vi "Process Standard Output.vi"(8 "error in (no error)":errorcluster, 11 "InsightCM Console Wrapper in":refnum<class "InsightCM Console Wrapper.lvclass">) -> (0 "error out":errorcluster, 2 "Command Output":string, 3 "InsightCM Console Wrapper out":refnum<class "InsightCM Console Wrapper.lvclass">)   [LabVIEW 2020, in "InsightCM Console Wrapper.lvclass"]
uses:
  InsightCM Console Wrapper.lvclass
  C:/Users/fflores/Documents/GitHub Projects/LabVIEW-CLI-Wrapper/Console Wrapper/Console Wrapper.lvclass
  Console Wrapper/Read Standard Output.vi
  <vilib>/Utility/error.llb/Error Cluster From Error Code.vi
  <vilib>/ErrorRing/Error Ring.xnode
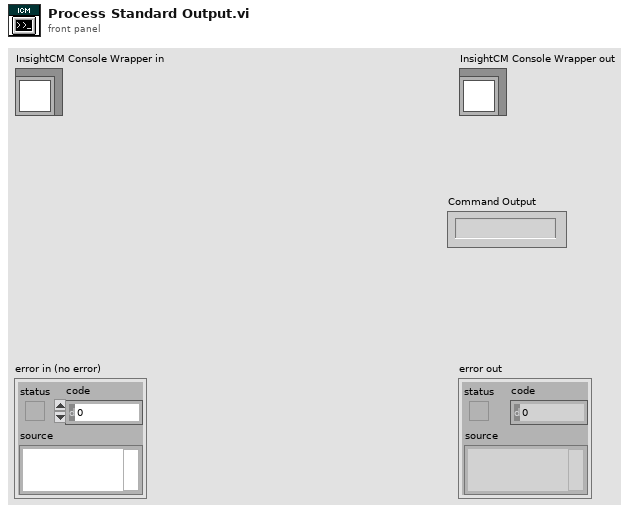
[diagram p1: front panel]
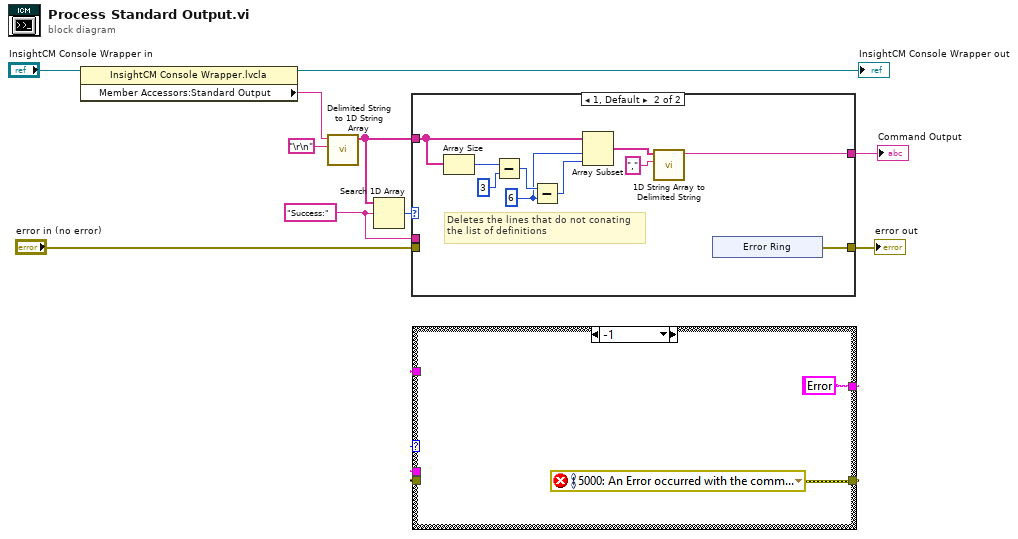
[diagram p0: block diagram]
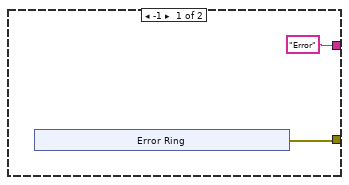
[diagram p2: hidden frame]
diagram:
  w5 = "Success:" ("element")
  n1 = property class="InsightCM Console Wrapper.lvcla"(reference="InsightCM Console Wrapper in") -> (reference out=→"InsightCM Console Wrapper out":refnum<class "InsightCM Console Wrapper.lvclass">, "Member Accessors:Standard Output"=w7:string)  [unwired: 1 in, 1 out]
  n2 = call <vilib>:"Delimited String to 1D String Array.vi"("delimiter"="\r\n", "delimited string"=w7) -> ("string array"=w6:string[])  [unwired: 9 in]
  n3 = Search 1D Array(1D array=w6, element=w5) -> (index of element=w4:i32)  [unwired: 1 in]
  n4 = case shown="1, Default" w4 {
    tunnel: "error in (no error)" -> [_ _]
    tunnel: w6 -> [_ w20]
    tunnel: [w12 w18] -> w1
    tunnel: w5 -> [_ _]
    tunnel: ["Error" ("delimited string") w19] -> w2
    frame -1 {
      n5 = xnode "Error Ring"() -> ("error out"=w12:errorcluster)
    }
    frame 1, Default {
      w21 = 6 ("y")
      # "Deletes the lines that do not conating\nthe list of definitions"
      n6 = Array Size(array=w20) -> (size(s)=w27:i32)
      n7 = Subtract(x=w27, y=3) -> (x-y=w25:i32)
      n8 = Subtract(x=w25, y=w21) -> (x-y=w26:i32)
      n9 = Array Subset(array=w20, index=w21, length=w26) -> (w24:string[])
      n10 = call <vilib>:"1D String Array to Delimited String.vi"("delimiter"=",", "string array"=w24) -> ("delimited string"=w19:string)  [unwired: 9 in]
      n11 = xnode "Error Ring"() -> ("error out"=w18:errorcluster)
    }
  }
  "error out" <- w1
  "Command Output" <- w2
